vi "Client_v1.vi"() -> ()   [LabVIEW 2019]
uses:
  <vilib>/LabVIEW Open Source Project/MQTT Client/Client class/Client.lvclass/Client.ctl
  <vilib>/LabVIEW Open Source Project/MQTT Connection/MQTT_Base/Base Class/MQTT_Base.lvclass/MQTT_Base.ctl
  <vilib>/LabVIEW Open Source Project/MQTT TCP Connection/MQTT_TCP/Connection/TCPConnection.lvclass
  C:/Program Files (x86)/National Instruments/LabVIEW 2019/vi.lib/LabVIEW Open Source Project/MQTT Connection/MQTT_Connection/Connection/Connection.lvclass
  <vilib>/LabVIEW Open Source Project/MQTT Client/Client class/Client.lvclass
  C:/Program Files (x86)/National Instruments/LabVIEW 2019/vi.lib/LabVIEW Open Source Project/MQTT Connection/MQTT_Base/Base Class/MQTT_Base.lvclass
  <vilib>/LabVIEW Open Source Project/MQTT Control Packets/Control Packets/PUBLISH/PUBLISH.lvclass
  <vilib>/LabVIEW Open Source Project/MQTT Connection/MQTT_Base/Base Class/MQTT_Base.lvclass
panel:
  in  "Period":i32
  in  "Connection":bool
  in  "Stop Client":bool
  out "Published":bool
  out "Waveform Chart":dbl(graph)
  out "last error":errorcluster
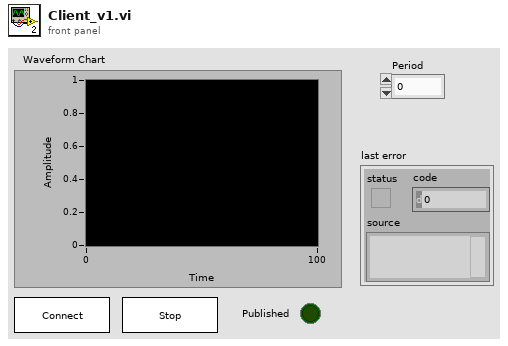
[diagram p1: front panel]
types:
  T1 = typedef "MQTT Client.lvlib/Client.lvclass/Public Events -- cluster.ctl" = cluster{"Connection Status":refnum<user-event>, "Connected":refnum<user-event>, "Application Message":refnum<user-event>}
  T2 = typedef "MQTT Base.lvlib/MQTT_Base.lvclass/Public Events -- cluster.ctl" = cluster{"Stop Event":refnum<user-event>, "Error Event":refnum<user-event>, "Inbound Message":refnum<user-event>}
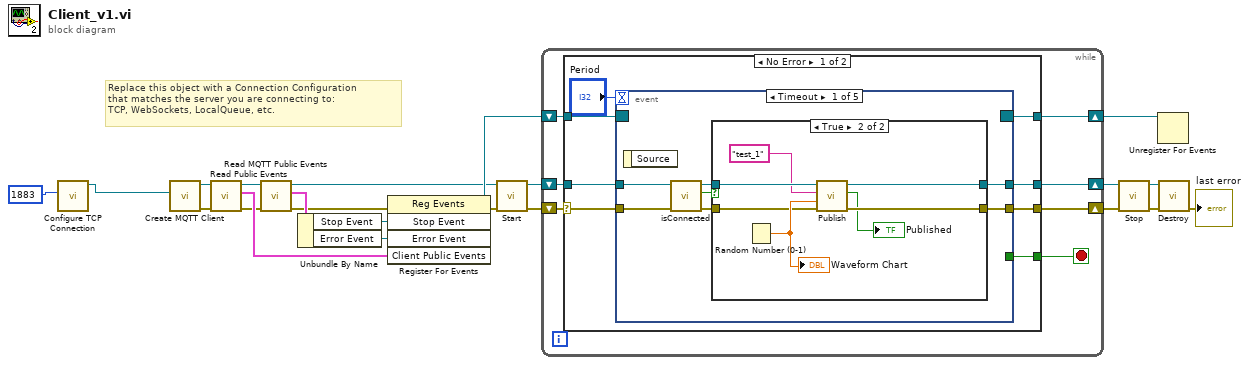
[diagram p0: block diagram]
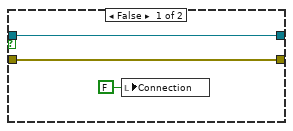
[diagram p2: hidden frame]
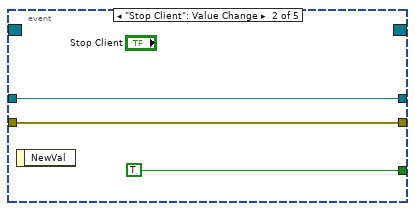
[diagram p3: hidden frame]
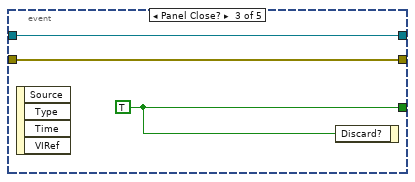
[diagram p4: hidden frame]
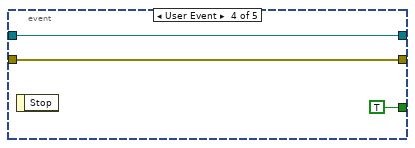
[diagram p5: hidden frame]
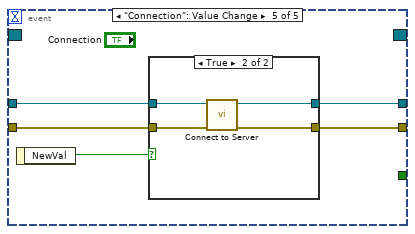
[diagram p6: hidden frame]
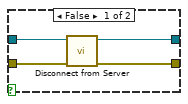
[diagram p7: hidden frame]
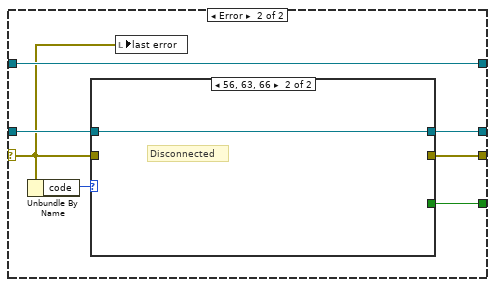
[diagram p8: hidden frame]
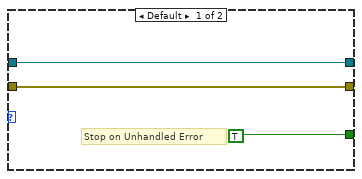
[diagram p9: hidden frame]
diagram:
  # "Replace this object with a Connection Configuration\nthat matches the server you are connecting to:\nTCP, WebSockets, LocalQueue, etc."
  n1 = call <vilib>:"Configure TCP Connection.vi"("remote port (80)"=u16 1883) -> ("TCPConnection"=w1:refnum<class "TCPConnection.lvclass">)  [unwired: 9 in, 1 out]
  n2 = call <vilib>:"Create MQTT Client.vi"("Connection Configuration"=w1) -> ("error out"=w5:errorcluster, "Client out"=w3:refnum<class "Client.lvclass">)  [unwired: 9 in]
  n3 = call <vilib>:"Read Public Events.vi"("error in (no error)"=w5, "Client in"=w3) -> ("error out"=w6:errorcluster, "Client Public Events"=w8:T1, "Client out"=w4:refnum<class "Client.lvclass">)  [unwired: 7 in]
  n4 = call <vilib>:"Read MQTT Public Events.vi"("error in (no error)"=w6, "MQTT_Base in"=w4) -> ("error out"=w7:errorcluster, "MQTT Public Events"=w15:T2, "MQTT_Base out"=w10:refnum<class "Client.lvclass">)  [unwired: 7 in]
  n5 = Unbundle By Name(w15) -> ("Stop Event"=w13:refnum<user-event>, "Error Event"=w14:refnum<user-event>)
  n6 = register-events(error in=w7, w13, w14, w8) -> (reference out=w11:refnum<event-registration>, error out=w9:errorcluster)  [unwired: 1 in]
  n7 = call <vilib>:"Start.vi"("error in (no error)"=w9, "MQTT_Base in"=w10) -> ("error out"=w21:errorcluster, "MQTT_Base out"=w20:refnum<class "Client.lvclass">)  [unwired: 7 in, 1 out]
  n8 = while {
    shift-right: [w28] -> w12
    shift-left: w11 -> [w29]
    shift-right: [w25] -> w17
    shift-left: w20 -> [w26]
    shift-right: [w27] -> w19
    shift-left: w21 -> [w23]
    stop <- w24 stop-if-true
    n9 = case shown="No Error" w23 {
      selector: w23 -> [w31 w77]
      tunnel: w29 -> [w37 w83]
      tunnel: [w36 w83] -> w28
      tunnel: [w35 w79] -> w27
      tunnel: w26 -> [w34 w81]
      tunnel: [w33 w80] -> w25
      tunnel: [w32 w78] -> w24
      frame No Error {
        n10 = event shown="[0] Timeout" {
          selector: w37 -> [_ _ _ _ _]
          dyn-events: [_ _ _ _ _] -> w36
          timeout: "Period" -> [_ _ _ _ _]
          tunnel: w31 -> [w40 w56 w58 w63 w64]
          tunnel: [w43 w56 w58 w63 w65] -> w35
          tunnel: [_ TRUE w60 TRUE _] -> w32
          tunnel: w34 -> [w42 w57 w59 w61 w68]
          tunnel: [w44 w57 w59 w61 w66] -> w33
          event Timeout {
            n11 = event-data() -> ()  [unwired: 1 in, 1 out]
            n12 = call <vilib>:"isConnected.vi"("error in (no error)"=w40, "Client in"=w42) -> ("error out"=w39:errorcluster, "connected"=w38:bool, "Client out"=w41:refnum<class "Client.lvclass">)  [unwired: 7 in]
            n13 = case shown="True" w38 {
              tunnel: [w47 w54] -> w44
              tunnel: [w46 w53] -> w43
              tunnel: w41 -> [w47 w50]
              tunnel: w39 -> [w46 w49]
              frame False {
                n14 = local write "Connection"(FALSE ("Connection")) -> ()
              }
              frame True {
                n15 = Random Number (0-1)() -> (number: 0 to 1=w51:dbl)
                "Waveform Chart" <- w51
                n16 = call <vilib>:"Publish.vi"("error in (no error)"=w49, "Payload"=w51, "Topic Name (empty: Payload name)"="test_1", "Client in"=w50) -> ("error out"=w53:errorcluster, "Published"=→"Published":bool, "Client out"=w54:refnum<class "Client.lvclass">)  [unwired: 5 in]
              }
            }
          }
          event "Stop Client": Value Change {
            n17 = event-data() -> ()  [unwired: 1 in, 1 out]
          }
          event Panel Close? {
            w60 = TRUE
            n18 = event-data() -> ()  [unwired: 1 in, 4 out]
            n19 = event-data("Discard?"=w60) -> ()  [unwired: 1 in, 1 out]
          }
          event User Event {
            n20 = event-data() -> ()  [unwired: 1 in, 1 out]
          }
          event "Connection": Value Change {
            n21 = event-data() -> ("NewVal"=w67:bool)  [unwired: 1 in]
            n22 = case shown="True" w67 {
              tunnel: w68 -> [w72 w76]
              tunnel: [w71 w73] -> w66
              tunnel: [w70 w74] -> w65
              tunnel: w64 -> [w69 w75]
              frame False {
                n23 = call <vilib>:"Disconnect from Server.vi"("error in (no error)"=w69, "Client in"=w72) -> ("error out"=w70:errorcluster, "Client out"=w71:refnum<class "Client.lvclass">)  [unwired: 7 in, 1 out]
              }
              frame True {
                n24 = call <vilib>:"Connect to Server.vi"("error in (no error)"=w75, "Client in"=w76) -> ("error out"=w74:errorcluster, "Client out"=w73:refnum<class "Client.lvclass">)  [unwired: 6 in, 2 out]
              }
            }
          }
        }
      }
      frame Error {
        n25 = Unbundle By Name(w77) -> ("code"=w82:i32)
        n26 = case shown="56, 63, 66" w82 {
          tunnel: w81 -> [w86 w87]
          tunnel: [w86 w87] -> w80
          tunnel: w77 -> [w85 _]
          tunnel: [w85 _] -> w79
          tunnel: [TRUE _] -> w78
          frame Default {
            # "Stop on Unhandled Error"
          }
          frame 56, 63, 66 {
            # "Disconnected"
          }
        }
        n27 = local write "last error"(w77) -> ()
      }
    }
  }
  n28 = call <vilib>:"Stop.vi"("error in (no error)"=w19, "MQTT_Base in"=w17) -> ("error out"=w18:errorcluster, "MQTT_Base out"=w16:refnum<class "Client.lvclass">)  [unwired: 7 in, 1 out]
  n29 = Unregister For Events(event registration refnum=w12) -> ()  [unwired: 1 in, 1 out]
  n30 = call <vilib>:"Destroy.vi"("error in (no error)"=w18, "MQTT_Base in"=w16) -> ("error out"=→"last error":errorcluster)  [unwired: 8 in, 1 out]
